vi "Connection Info.vi"() -> (2 "Connection Count":i32, 3 "Connected":bool)   [LabVIEW 2025]
doc: "Return basic information about Network Table Connections."
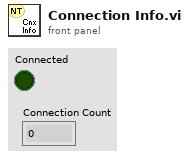
[diagram p1: front panel]
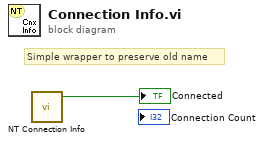
[diagram p0: block diagram]
diagram:
  # "Simple wrapper to preserve old name"
  n1 = call <vilib>:"NT Connection Info.vi"() -> ("Connected"=→"Connected":bool)  [unwired: 11 in]
